vi "String array concatenation.vi"(1 "Above?":bool, 2 "Add End of Line?":bool, 3 "Array of Strings":string[](array[string]), 4 "Input String":string) -> (0 "Concatenated Array":string)   [LabVIEW 2011]
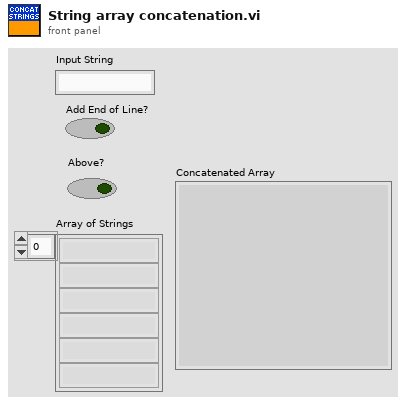
[diagram p1: front panel]
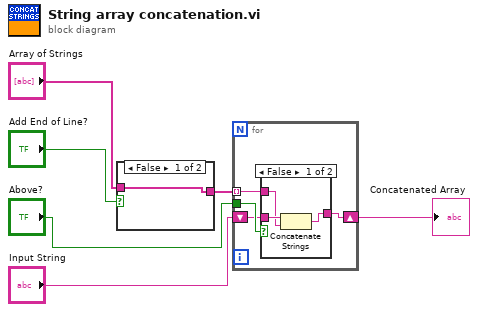
[diagram p0: block diagram]
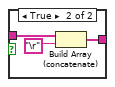
[diagram p2: hidden frame]
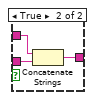
[diagram p3: hidden frame]
diagram:
  n1 = case shown="False" "Add End of Line?" {
    tunnel: "Array of Strings" -> [w7 w9]
    tunnel: [w7 w8] -> w1
    frame False {
    }
    frame True {
      n2 = Build Array (concatenate)(w9, "\r") -> (w8:string[])
    }
  }
  n3 = for {
    tunnel: w1 -> [w11] mode=indexing
    shift-right: [w14] -> w5
    shift-left: "Input String" -> [w12]
    tunnel: "Above?" -> [w13]
    n4 = case shown="False" w13 {
      tunnel: [w17 w20] -> w14
      tunnel: w12 -> [w16 w19]
      tunnel: w11 -> [w15 w18]
      frame False {
        n5 = Concatenate Strings(w16, w15) -> (w17:string)
      }
      frame True {
        n6 = Concatenate Strings(w18, w19) -> (w20:string)
      }
    }
  }
  "Concatenated Array" <- w5
